vi "Threshold with Hysteresis 2012 NIVerified.vi"(8 "Hysteresis":dbl, 9 "Threshold":dbl, 10 "Boolean 2":bool, 11 "signal in":dbl) -> (1 "Peak":i32)   [LabVIEW 2012]
doc: "Use this template to build a standard state machine design pattern. Each state executes code and determines which state to transition to. Contrast this design pattern with the User Interface Event Handler pattern, in which code executes in response to user actions. Contrast this design pattern also with the Queued Message Handler pattern, in which each message handling code can queue zero or more new messages."
uses:
  peak w hysteresis.ctl
panel:
  out "Boolean":bool
  out "comparator":dbl
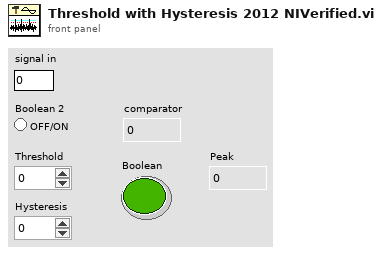
[diagram p1: front panel]
types:
  T1 = typedef "peak w hysteresis.ctl" = enum16{"Wait", "Peak", "Repeat?", "Stop"}
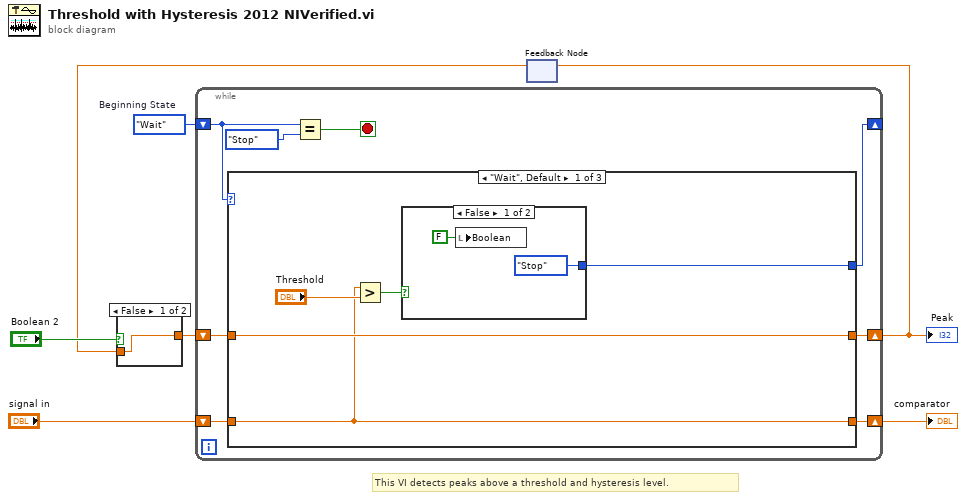
[diagram p0: block diagram]
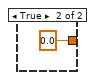
[diagram p2: hidden frame]
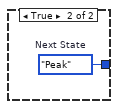
[diagram p3: hidden frame]
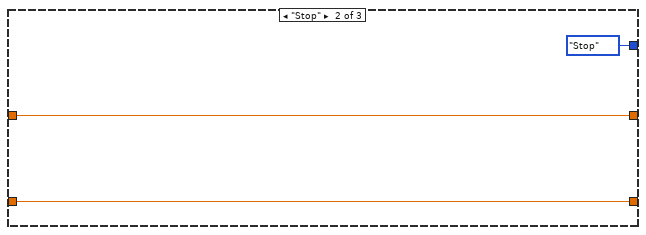
[diagram p4: hidden frame]
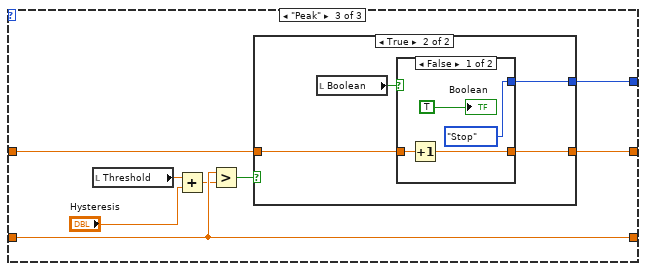
[diagram p5: hidden frame]
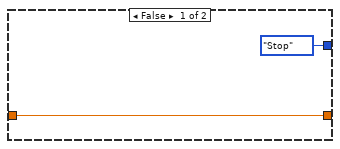
[diagram p6: hidden frame]
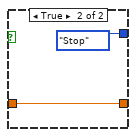
[diagram p7: hidden frame]
diagram:
  w7 = peak_w_hysteresis."Wait"  # Beginning State
  # "This VI detects peaks above a threshold and hysteresis level."
  n1 = feedback #1() -> (w1:dbl)  [unwired: 1 in]
  n2 = case shown="False" "Boolean 2" {
    tunnel: [w8 0.0] -> w5
    tunnel: w1 -> [w8 _]
    frame False {
    }
    frame True {
    }
  }
  n3 = while {
    shift-right: [w14] -> _
    shift-left: w7 -> [w15]
    shift-right: [w10] -> w6
    shift-left: "signal in" -> [w13]
    shift-right: [w11] -> w2
    shift-left: w5 -> [w12]
    stop <- w17 stop-if-true
    n4 = case shown="\"Wait\", Default" w15 {
      tunnel: [w22 peak_w_hysteresis."Stop" ("Next State") w33] -> w14
      tunnel: w13 -> [w18 w27 w34]
      tunnel: [w18 w27 w34] -> w10
      tunnel: w12 -> [w19 w26 w36]
      tunnel: [w19 w26 w35] -> w11
      frame "Wait", Default {
        n5 = Greater?(x=w18, y="Threshold") -> (0:w21:bool)
        n6 = case shown="False" w21 {
          tunnel: [peak_w_hysteresis."Stop" ("Next State") w25] -> w22
          frame False {
            n7 = local write "Boolean"(FALSE ("Boolean")) -> ()
          }
          frame True {
            w25 = peak_w_hysteresis."Peak"  # Next State
          }
        }
      }
      frame "Stop" {
      }
      frame "Peak" {
        n8 = local read "Threshold"() -> (w30:dbl)
        n9 = Add(x=w30, y="Hysteresis") -> (x+y=w31:dbl)
        n10 = Greater?(x=w34, y=w31) -> (0:w32:bool)
        n11 = case shown="True" w32 {
          tunnel: w36 -> [w38 w42]
          tunnel: [w38 w41] -> w35
          tunnel: [peak_w_hysteresis."Stop" ("Next State") w40] -> w33
          frame False {
          }
          frame True {
            n12 = local read "Boolean"() -> (w39:bool)
            n13 = case shown="False" w39 {
              tunnel: w42 -> [w45 w47]
              tunnel: [w44 w47] -> w41
              tunnel: [peak_w_hysteresis."Stop" ("Next State") peak_w_hysteresis."Stop" ("Next State")] -> w40
              frame False {
                n14 = Increment(x=w45) -> (x+1=w44:dbl)
                "Boolean" <- TRUE ("Boolean")
              }
              frame True {
              }
            }
          }
        }
      }
    }
    n15 = Equal?(x=w15, y=peak_w_hysteresis."Stop" ("States")) -> (x = y?=w17:bool)
  }
  "Peak" <- w2
  "comparator" <- w6
  n16 = feedback-in #1(w2) -> ()
